vi "eval Comm.vi"(8 "error in (no error)":errorcluster caption="Fehler (Eingang, kein Fehler)", 10 "Commandline":string, 11 "TestInterface Eingang":refnum<class "TestInterface.lvclass"> caption="DNL_LabVIEW Object in") -> (0 "error out":errorcluster caption="Fehler (Ausgang)", 1 "isQuerry":bool, 2 "timeout(ms)":i32, 3 "TestInterface Ausgang":refnum<class "TestInterface.lvclass"> caption="DNL_LabVIEW Object out")   [LabVIEW 2013]
uses:
  TestInterface.lvclass
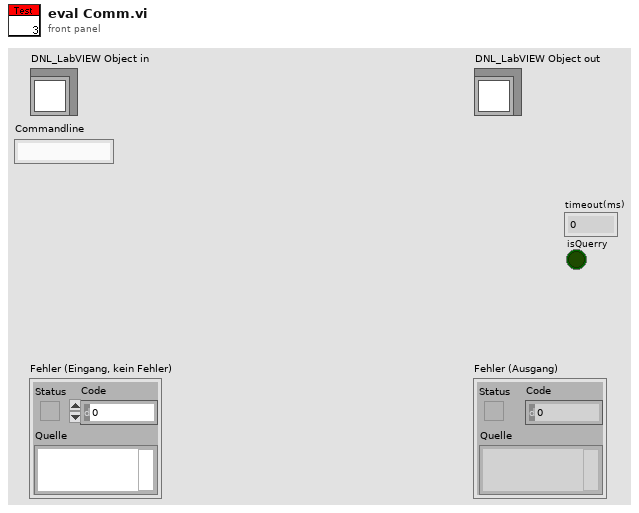
[diagram p1: front panel]
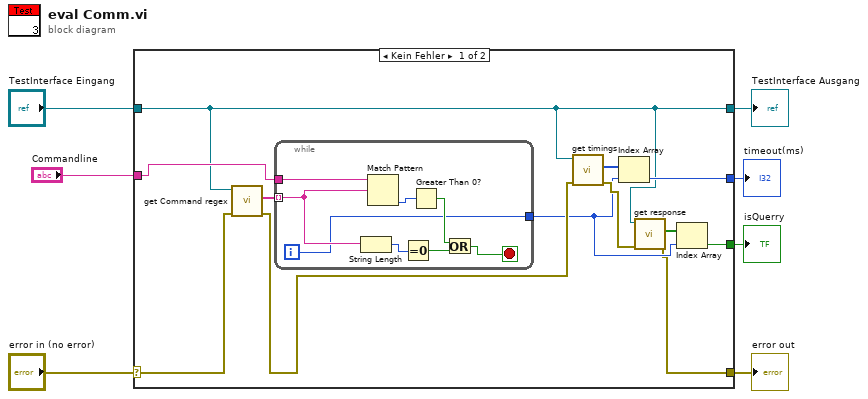
[diagram p0: block diagram]
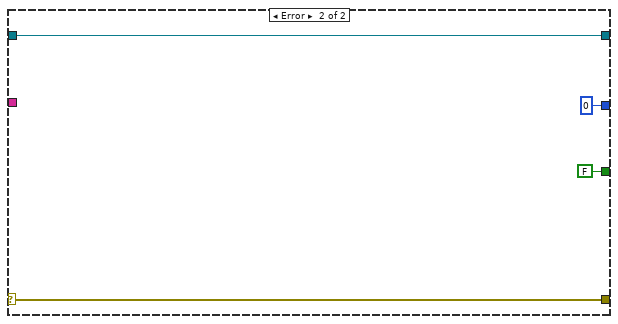
[diagram p2: hidden frame]
diagram:
  n1 = case shown="Kein Fehler" "error in (no error)" {
    selector: "error in (no error)" -> [w17 w31]
    tunnel: [w9 w31] -> w6
    tunnel: [w13 w30] -> w4
    tunnel: "TestInterface Eingang" -> [w13 w30]
    tunnel: "Commandline" -> [w19 _]
    tunnel: [w14 0 ("Numerisch")] -> w2
    tunnel: [w8 FALSE ("Boolesch")] -> w1
    frame No Error {
      n2 = call-dynamic "get Command regex.vi"("error in (no error)"=w17, "TestInterface (Eingang)"=w13) -> ("error out"=w16:errorcluster, "Command regex"=w18:string[])  [unwired: 7 in, 1 out]
      n3 = while {
        tunnel: w19 -> [w27]
        tunnel: w18 -> [w25] mode=indexing
        tunnel: [w20] -> w10
        i -> [w20]
        stop <- w23 stop-if-true
        n4 = String Length(string=w25) -> (length=w26:i32)
        n5 = Match Pattern(string=w27, regular expression=w25) -> (offset past match=w22:i32)  [unwired: 1 in, 3 out]
        n6 = Equal To 0?(x=w26) -> (x = 0?=w24:bool)
        n7 = Greater Than 0?(x=w22) -> (x > 0?=w21:bool)
        n8 = Or(x=w21, y=w24) -> (x .or. y?=w23:bool)
      }
      n9 = call-dynamic "get timings.vi"("error in (no error)"=w16, "TestInterface (Eingang)"=w13) -> ("error out"=w12:errorcluster, "timings"=w15:i32[])  [unwired: 7 in, 1 out]
      n10 = Index Array(array=w15, index=w10) -> (element=w14:i32)
      n11 = call-dynamic "get response.vi"("error in (no error)"=w12, "TestInterface (Eingang)"=w13) -> ("error out"=w9:errorcluster, "response?"=w11:bool[])  [unwired: 7 in, 1 out]
      n12 = Index Array(array=w11, index=w10) -> (element=w8:bool)
    }
    frame Error {
    }
  }
  "error out" <- w6
  "TestInterface Ausgang" <- w4
  "timeout(ms)" <- w2
  "isQuerry" <- w1
